vi "Create Sub Vi.vi"() -> ()   [LabVIEW 2020]
panel:
  in  "Numeric 2":i32
  out "Factorial":i32
  # "Factorial Sub VI"
  # "1x1 =1\n2x1 =2\n2x3 =6\n6x4 =24\n24x5 =125"
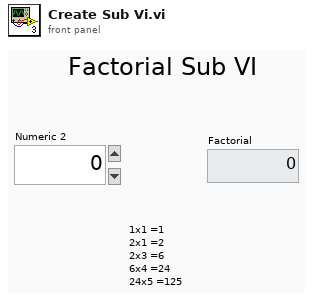
[diagram p1: front panel]
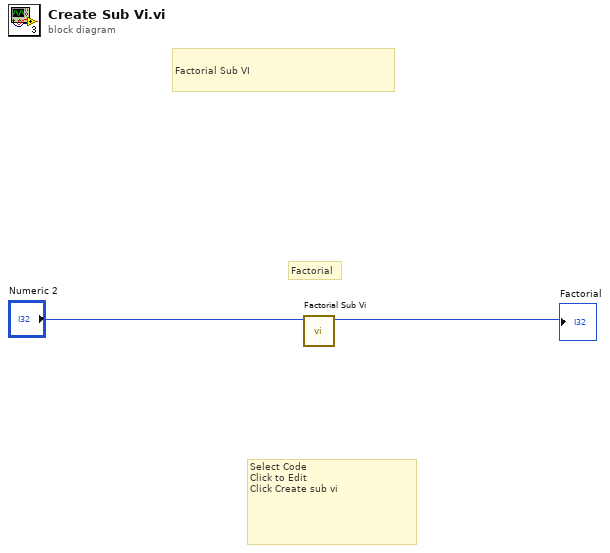
[diagram p0: block diagram]
diagram:
  # "Factorial"
  # "Select Code\nClick to Edit\nClick Create sub vi"
  # "Factorial Sub VI"
  n1 = call "Factorial Sub Vi.vi"("Numeric in"="Numeric 2") -> ("Numeric out"=→"Factorial":i32)  [unwired: 10 in]
